vi "Validate User (SubVI).vi"(11 "App Data":T1) -> (2 "Exit?":bool, 3 "User Data":T2 {"UserType" items=["Admin", "Operator"]})   [LabVIEW 2021]
uses:
  Controls/UserTypes.ctl
  Controls/UserData.ctl
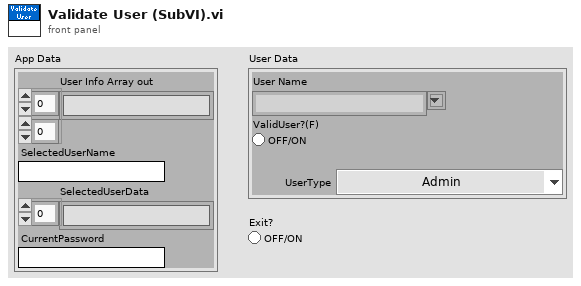
[diagram p1: front panel]
types:
  T1 = cluster{"User Info Array out":string[][], "SelectedUserName":string, "SelectedUserData":string[], "CurrentPassword":string}
  T2 = typedef "UserData.ctl" = cluster{"User Name":string, "ValidUser?(F)":bool, "UserType":T3}
  T3 = typedef "UserTypes.ctl" = u16
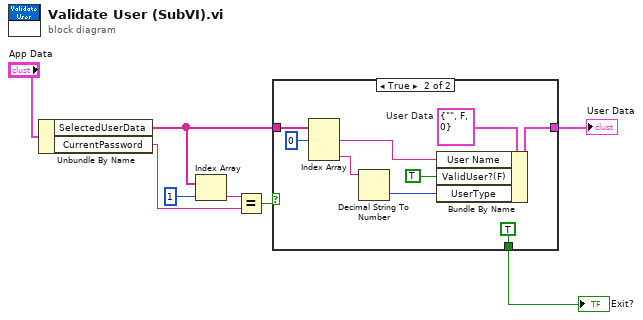
[diagram p0: block diagram]
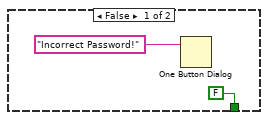
[diagram p2: hidden frame]
diagram:
  n1 = Unbundle By Name("App Data") -> ("SelectedUserData"=w7:string[], "CurrentPassword"=w3:string)
  n2 = Index Array(array=w7, index=1) -> (element=w2:string)
  n3 = Equal?(x=w2, y=w3) -> (x = y?=w6:bool)
  n4 = case shown="True" w6 {
    tunnel: [_ w18] -> w5
    tunnel: w7 -> [_ w17]
    tunnel: [FALSE ("ValidUser?(F)") TRUE ("ValidUser?(F)")] -> w8
    frame False {
      n5 = One Button Dialog(message="Incorrect Password!") -> ()  [unwired: 1 in, 1 out]
    }
    frame True {
      w19 = T2 {"User Name"="", "ValidUser?(F)"=FALSE, "UserType"=0}  # User Data
      n6 = Index Array(array=w17, index #1=0 ("index")) -> (element #1=w15:string, element #3=w13:string)  [unwired: 2 in, 1 out]
      n7 = Decimal String To Number(string=w13) -> (number=w12:i32)  [unwired: 2 in, 1 out]
      n8 = Bundle By Name(cluster=w19, "User Name"=w15, "ValidUser?(F)"=TRUE, "UserType"=w12) -> (w18:T2)
    }
  }
  "Exit?" <- w8
  "User Data" <- w5
